vi "Progress.vi"(8 "error in (no error)":errorcluster, 9 "Progress (%)":i32, 10 "Message":string, 11 "StartupSplash in":refnum<class "StartupSplash.lvclass">) -> (0 "error out":errorcluster, 3 "StartupSplash out":refnum<class "StartupSplash.lvclass">)   [LabVIEW 2025, in "StartupSplash.lvclass"]
uses:
  StartupSplash.lvclass
  StartupSplash.lvclass/StartupSplash.ctl
  zeromq/Send_string.vi
  zeromq/Socket.lvclass
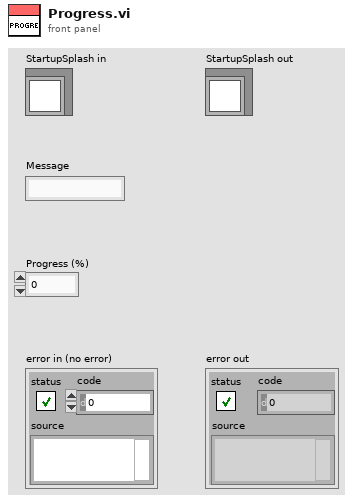
[diagram p1: front panel]
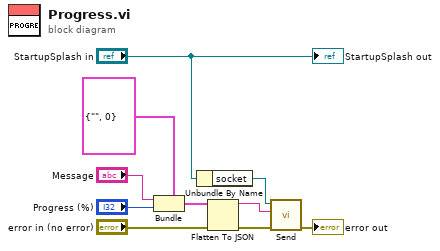
[diagram p0: block diagram]
diagram:
  n1 = Bundle(cluster=cluster{"status":string, "progress":i32} {"status"="", "progress"=0}, "status"="Message", "progress"="Progress (%)") -> (w7:cluster{"status":string, "progress":i32})
  n2 = Unbundle By Name("StartupSplash in") -> ("socket"=w4:refnum<class "Socket.lvclass">)
  n3 = Flatten To JSON(anything=w7, error in (no error)="error in (no error)") -> (JSON string=w3:string, 11:w2:errorcluster)  [unwired: 1 in]
  n4 = call-poly "Send.vi"("error in"=w2, "data"=w3, "socket in"=w4) -> ("error out"=→"error out":errorcluster)  [unwired: 7 in, 1 out]
  "StartupSplash out" <- "StartupSplash in"
